vi "Get Metadata.vi"() -> (4 "shared metadata":T1)   [LabVIEW 2025, in "niUSRP Rx Core v1 FPGA.lvclass"]
uses:
  niUSRP Rx Core v1 FPGA.lvclass
  <instrlib>/_niInstr/Instruction Framework/v1/FPGA/Collection Builder/Parent Metadata.ctl
  <instrlib>/_niInstr/Instruction Framework/v1/FPGA/Collection Builder/niInstr Address Space Collection Builder v1 FPGA.lvlib
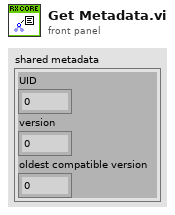
[diagram p1: front panel]
types:
  T1 = typedef "niInstr Address Space Collection Builder v1 FPGA.lvlib/Parent Metadata.ctl" = cluster{"UID":u16, "version":u16, "oldest compatible version":u16}
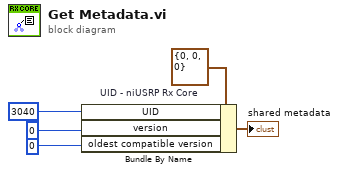
[diagram p0: block diagram]
diagram:
  w4 = u16 3040  # UID - niUSRP Rx Core
  n1 = Bundle By Name(cluster=T1 {"UID"=0, "version"=0, "oldest compatible version"=0} ("parent metadata"), "UID"=w4, "version"=u16 0, "oldest compatible version"=u16 0) -> (→"shared metadata":T1)
